vi "Read PID.vi"(8 "error in (no error)":errorcluster, 11 "Humidity Control in":refnum<class "Humidity Control.lvclass">) -> (0 "error out":errorcluster, 2 "PID":cluster{"P":dbl, "I":dbl, "D":dbl}, 3 "Humidity Control out":refnum<class "Humidity Control.lvclass">)   [LabVIEW 2015, in "Humidity Control.lvclass"]
uses:
  Humidity Control.lvclass
  Humidity Control.lvclass/Humidity Control.ctl
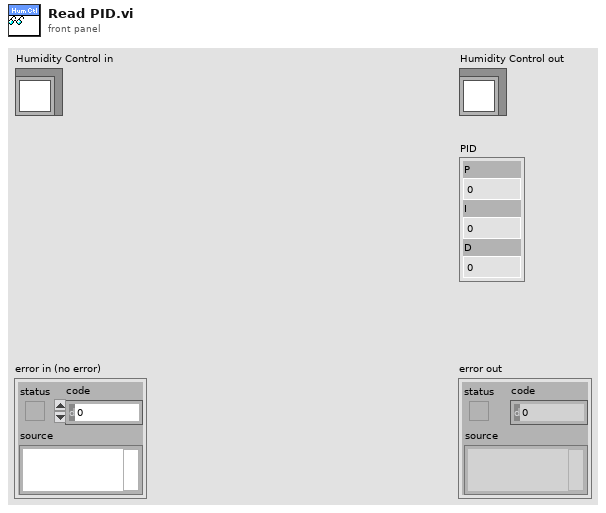
[diagram p1: front panel]
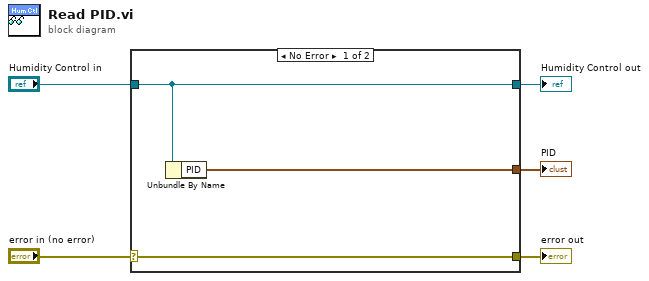
[diagram p0: block diagram]
diagram:
  n1 = case shown="No Error" "error in (no error)" {
    selector: "error in (no error)" -> [w8 w9]
    tunnel: [w8 w9] -> w4
    tunnel: [w7 w10] -> w2
    tunnel: "Humidity Control in" -> [w7 w10]
    tunnel: [w6 _] -> w1
    frame No Error {
      n2 = Unbundle By Name(w7) -> ("PID"=w6:cluster{"P":dbl, "I":dbl, "D":dbl})
    }
    frame Error {
    }
  }
  "error out" <- w4
  "Humidity Control out" <- w2
  "PID" <- w1
